vi "TryDeleteWaveform.vi"(3 "error in (no error)":errorcluster, 4 "Waveform Name":string="WfmImport", 5 "VISA resource name":refnum<visa-resource-name>) -> (0 "error out":errorcluster, 1 "Waveform Deleted":bool, 2 "VISA resource name out":refnum<visa-resource-name>)   [LabVIEW 2020, in "Active Technologies AWG3000.lvlib"]
uses:
  Active Technologies AWG3000.lvlib
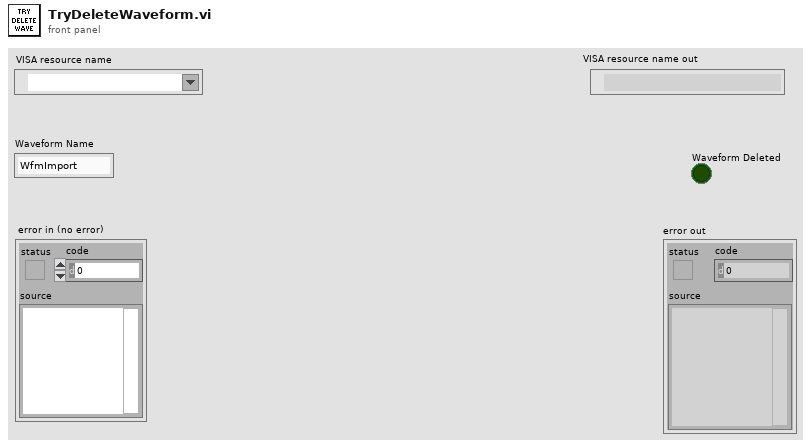
[diagram p1: front panel]
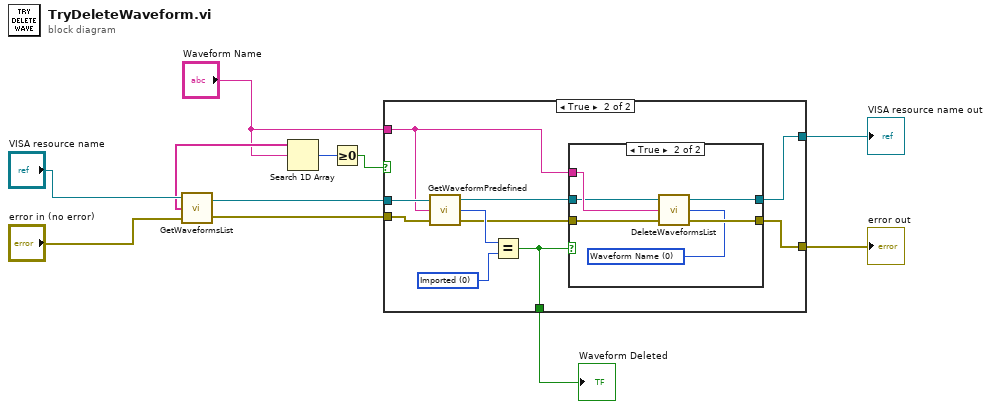
[diagram p0: block diagram]
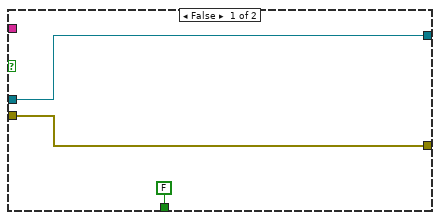
[diagram p2: hidden frame]
diagram:
  n1 = call "GetWaveformsList.vi"("error in (no error)"="error in (no error)", "VISA resource name"="VISA resource name") -> ("error out"=w7:errorcluster, "VISA resource name out"=w8:refnum<visa-resource-name>, "Waveforms List"=w9:string[])
  n2 = Search 1D Array(1D array=w9, element="Waveform Name") -> (index of element=w3:i32)  [unwired: 1 in]
  n3 = Greater Or Equal To 0?(x=w3) -> (x >= 0?=w2:bool)
  n4 = case shown="True" w2 {
    tunnel: w8 -> [w14 w22]
    tunnel: w7 -> [w13 w21]
    tunnel: "Waveform Name" -> [_ w20]
    tunnel: [w14 w24] -> w5
    tunnel: [w13 w23] -> w4
    tunnel: [FALSE w15] -> w1
    frame False {
    }
    frame True {
      w19 = u16 0 items=["Imported", "Predefined"] ("Waveform Type")
      n5 = call "GetWaveformPredefined.vi"("error in (no error)"=w21, "Waveform Name"=w20, "VISA resource name"=w22) -> ("error out"=w16:errorcluster, "Waveform Type"=w18:u16, "VISA resource name out"=w17:refnum<visa-resource-name>)
      n6 = Equal?(x=w18, y=w19) -> (x = y?=w15:bool)
      n7 = case shown="True" w15 {
        tunnel: [w26 w27] -> w24
        tunnel: [w25 w32] -> w23
        tunnel: w20 -> [_ w30]
        tunnel: w17 -> [w26 w29]
        tunnel: w16 -> [w25 w28]
        frame False {
        }
        frame True {
          w31 = u16 0 items=["Waveform Name", "All (Only Imported Waveforms)"] ("Delete Waveform Options")
          n8 = call "DeleteWaveformsList.vi"("Delete Waveform Options"=w31, "error in (no error)"=w28, "Delete Waveform from Waveform List (Name)"=w30, "VISA resource name"=w29) -> ("error out"=w32:errorcluster, "VISA resource name out"=w27:refnum<visa-resource-name>)
        }
      }
    }
  }
  "VISA resource name out" <- w5
  "error out" <- w4
  "Waveform Deleted" <- w1
